vi "AcquireImages.vi"(8 "Error In":errorcluster, 9 "Acquisition Parameters":T5={"Acquisition Mode"=enum."Single Scan", "Trigger Mode"=enum."Internal", "Frame \nTransfer"=FALSE, "Exposure Time (s)"=0.0, "Accumulation Cycle Time (s)"=0.0, "# Accumulations"=1, "# Kinetics"=1, "Kinetic Cycle Time (s)"=0.0, "Horizontal Bin Size"=1, "Vertical Bin Size"=1} {"Vertical Bin Size" min=1; "Horizontal Bin Size" min=1; "Kinetic Cycle Time (s)" format="%.2f"; "# Kinetics" min=1; "# Accumulations" min=1; "Accumulation Cycle Time (s)" format="%.2f"; "Exposure Time (s)" format="%.2e"}, 10 "Camera Information 2":T1 {"VS Speed (us)" format="%.2f"}, 11 "Pre Initialized?":bool) -> (0 "error out":errorcluster, 1 "Intensity Graph":i32[][](graph))   [LabVIEW 2013]
uses:
  camera_controls.ctl
  <userlib>/atmcd32d.llb/AcquisitionMode_mode typedef.ctl
  <userlib>/atmcd32d.llb/TriggerMode_mode typedef.ctl
  acquisition_states.ctl
  CameraTest/System Files/user.lib/atmcd32d.llb/Error Code Enum typedef.ctl
panel:
  out "Total Number Pixels":dbl format="%#_6f"
  out "Img Y Size":dbl
  out "Img X Size":dbl
  out "size(s)":i32[](array[numeric])
  out "# Acq'd Images":u32
  out "1D Images":i32[](array[numeric])
  out "Acq. Error Codes":T2
  out "Calcualted Times":T3 {"Kinetic" format="%.2f"; "Accumulate" format="%.2f"; "Exposure" format="%.2f"}
  out "Andor Initialization Error Codes":T4
  out "Camera Information":T1 {"VS Speed (us)" format="%.2f"}
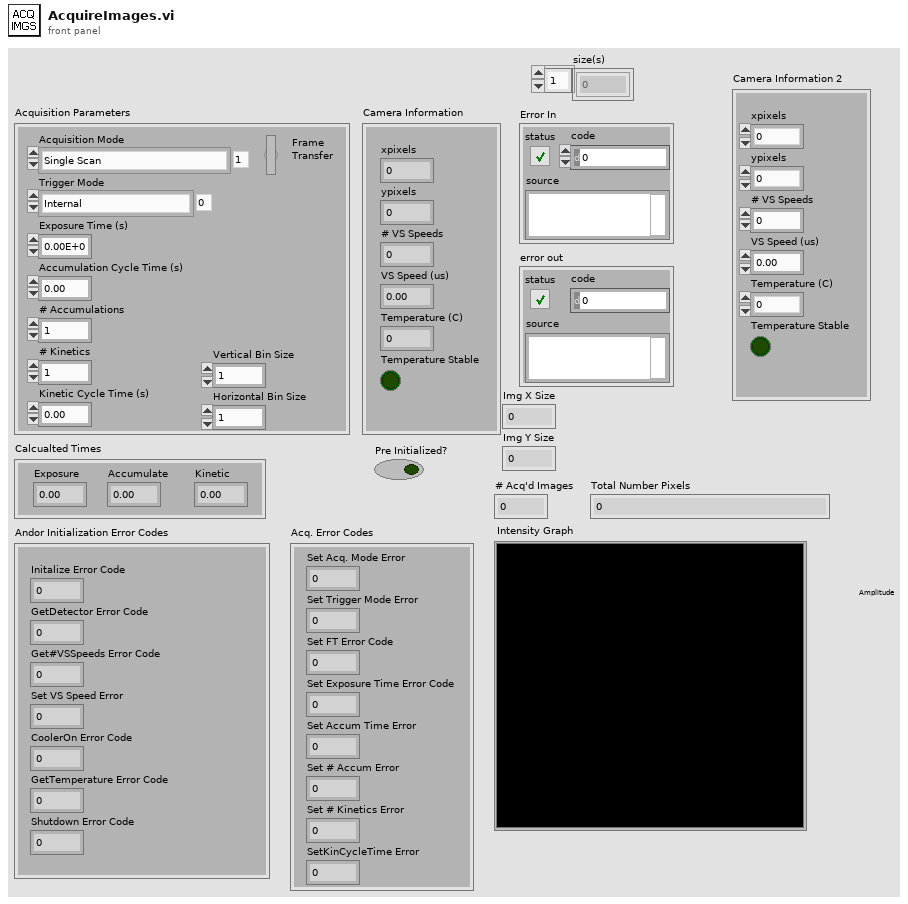
[diagram p1: front panel]
types:
  T1 = cluster{"xpixels":i32, "ypixels":i32, "# VS Speeds":i32, "VS Speed (us)":sgl, "Temperature Stable":bool, "Temperature (C)":i32}
  T2 = cluster{"Set Acq. Mode Error":u32, "Set Trigger Mode Error":u32, "Set FT Error Code":u32, "Set Exposure Time Error Code":u32, "Set Accum Time Error":u32, "Set # Accum Error":u32, "Set # Kinetics Error":u32, "SetKinCycleTime Error":u32}
  T3 = cluster{"Exposure":sgl, "Accumulate":sgl, "Kinetic":sgl}
  T4 = cluster{"Initalize Error Code":u32, "GetDetector Error Code":u32, "Get#VSSpeeds Error Code":u32, "Set VS Speed Error":u32, "CoolerOn Error Code":u32, "GetTemperature Error Code":u32, "Shutdown Error Code":u32}
  T5 = typedef "camera_controls.ctl" = cluster{"Acquisition Mode":T6, "Trigger Mode":T7, "Frame \nTransfer":bool, "Exposure Time (s)":sgl, "Accumulation Cycle Time (s)":sgl, "# Accumulations":i32, "# Kinetics":i32, "Kinetic Cycle Time (s)":sgl, "Horizontal Bin Size":i32, "Vertical Bin Size":i32}
  T6 = typedef "AcquisitionMode_mode typedef.ctl" = enum16{"Reserved (0)", "Single Scan", "Accumulate", "Kinetics", "Fast Kinetics", "Run Till Abort", "Reserved (6)", "Reserved (7)", "Reserved (8)", "Time Delayed Integration"}
  T7 = typedef "TriggerMode_mode typedef.ctl" = enum16{"Internal", "External", "N/A (2)", "N/A (3)", "N/A (4)", "N/A (5)", "External Start", "External Exposure (Bulb)", "N/A (8)", "External FVB EM", "Software", "N/A (11)", "External Charge Shifting"}
  T8 = typedef "acquisition_states.ctl" = enum16{"Initialize", "Set Params", "Begin Acquisition", "Retrive Data", "Display Data"}
  T9 = typedef "Error Code Enum typedef.ctl" = enum32{"N/A (0)", "DRV_ERROR_CODES", "DRV_SUCCESS", "DRV_VXDNOTINSTALLED", "DRV_ERROR_SCAN", "DRV_ERROR_CHECK_SUM", "DRV_ERROR_FILELOAD", "DRV_UNKNOWN_FUNC", "DRV_ERROR_VXD_INIT", "DRV_ERROR_ADDRESS", "DRV_ERROR_PAGELOCK", "DRV_ERROR_PAGEUNLOCK", "DRV_ERROR_BOARDTEST", "DRV_ERROR_ACK", "DRV_ERROR_UP_FIFO", "DRV_ERROR_PATTERN", "N/A (16)", "DRV_ACQUISITION_ERRORS", "DRV_ACQ_BUFFER", "DRV_ACQ_DOWNFIFO_FULL", "DRV_PROC_UNKONWN_INSTRUCTION", "DRV_ILLEGAL_OP_CODE", "DRV_KINETIC_TIME_NOT_MET", "DRV_ACCUM_TIME_NOT_MET", "DRV_NO_NEW_DATA", "N/A (25)", "DRV_SPOOLERROR", "N/A (27)", "N/A (28)", "N/A (29)", "N/A (30)", "N/A (31)", "N/A (32)", "DRV_TEMPERATURE_CODES", "DRV_TEMPERATURE_OFF", "DRV_TEMPERATURE_NOT_STABILIZED", "DRV_TEMPERATURE_STABILIZED", "DRV_TEMPERATURE_NOT_REACHED", "DRV_TEMPERATURE_OUT_RANGE", "DRV_TEMPERATURE_NOT_SUPPORTED", "DRV_TEMPERATURE_DRIFT", "N/A (41)", "N/A (42)", "N/A (43)", "N/A (44)", "N/A (45)", "N/A (46)", "N/A (47)", "N/A (48)", "DRV_GENERAL_ERRORS", "DRV_INVALID_AUX", "DRV_COF_NOTLOADED", "DRV_FPGAPROG", "DRV_FLEXERROR", "DRV_GPIBERROR", "N/A (55)", "N/A (56)", "N/A (57)", "N/A (58)", "N/A (59)", "N/A (60)", "N/A (61)", "N/A (62)", "N/A (63)", "DRV_DATATYPE", "DRV_DRIVER_ERRORS", "DRV_P1INVALID", "DRV_P2INVALID", "DRV_P3INVALID", "DRV_P4INVALID", "DRV_INIERROR", "DRV_COFERROR", "DRV_ACQUIRING", "DRV_IDLE", "DRV_TEMPCYCLE", "DRV_NOT_INITIALIZED", "DRV_P5INVALID", "DRV_P6INVALID", "DRV_INVALID_MODE", "DRV_INVALID_FILTER", "DRV_I2CERRORS", "DRV_I2CDEVNOTFOUND", "DRV_I2CTIMEOUT", "DRV_P7INVALID", "N/A (84)", "N/A (85)", "N/A (86)", "N/A (87)", "N/A (88)", "N/A (89)", "DRV_IOCERROR", "DRV_VRMVERSIONERROR"}
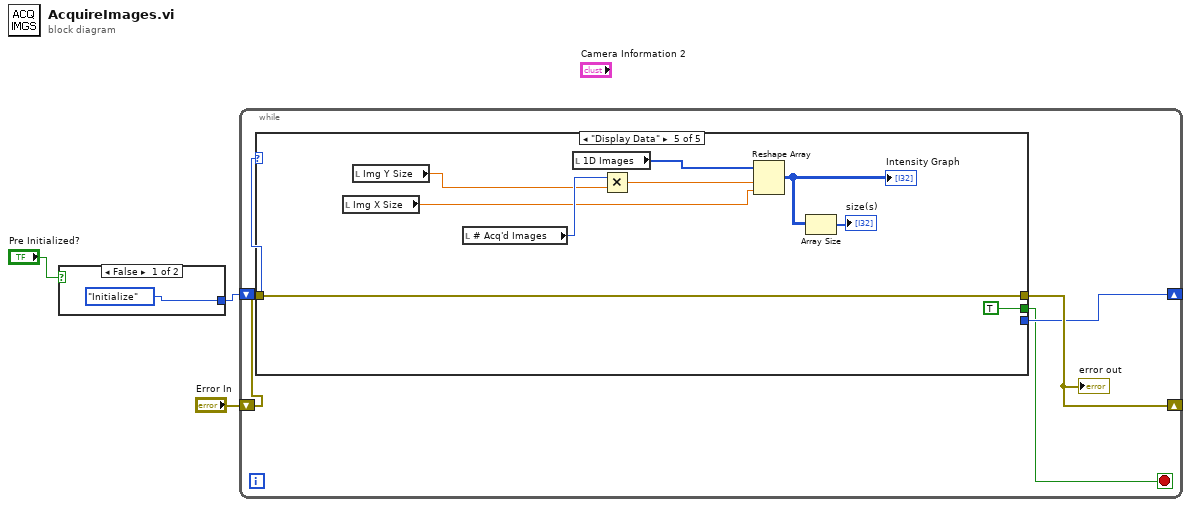
[diagram p0: block diagram]
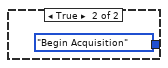
[diagram p2: hidden frame]
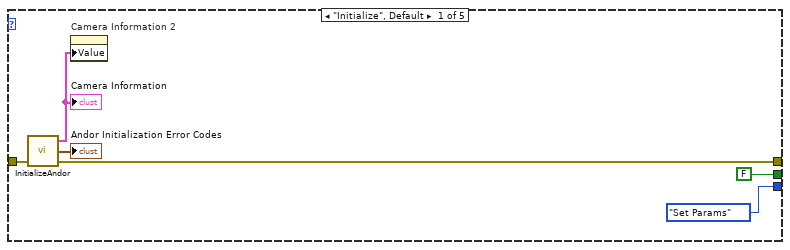
[diagram p3: hidden frame]
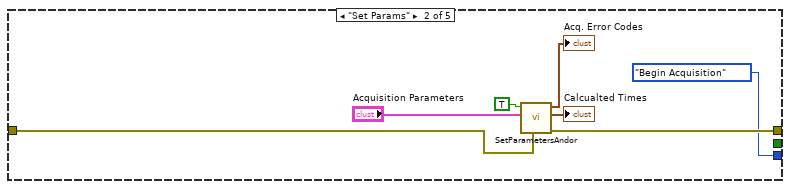
[diagram p4: hidden frame]
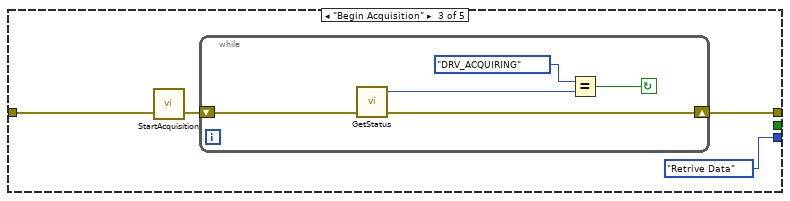
[diagram p5: hidden frame]
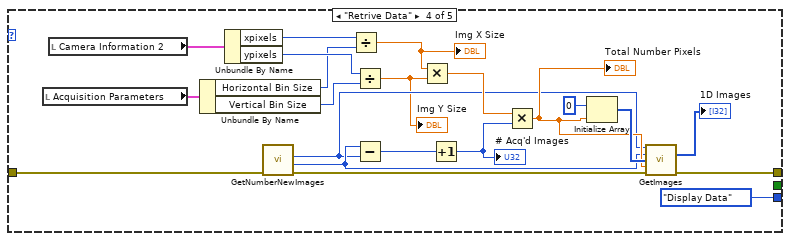
[diagram p6: hidden frame]
diagram:
  n1 = case shown="False" "Pre Initialized?" {
    tunnel: [acquisition_states."Initialize" acquisition_states."Begin Acquisition"] -> w3
    frame False {
    }
    frame True {
    }
  }
  n2 = while {
    shift-right: [w8] -> _
    shift-left: "Error In" -> [w9]
    shift-right: [w7] -> _
    shift-left: w3 -> [w10]
    stop <- w6 stop-if-true
    n3 = case shown="\"Display Data\"" w10 {
      tunnel: w9 -> [w16 w21 w27 w53 w60]
      tunnel: [w15 w20 w25 w47 w60] -> w8
      tunnel: [acquisition_states."Set Params" acquisition_states."Begin Acquisition" acquisition_states."Retrive Data" acquisition_states."Display Data" _] -> w7
      tunnel: [FALSE _ _ _ TRUE] -> w6
      frame "Initialize", Default {
        n4 = call "InitializeAndor.vi"("Error In"=w16) -> ("error out"=w15:errorcluster, "Andor Initialization Error Codes"=→"Andor Initialization Error Codes":T4, "Camera Information"=w11:T1)  [unwired: 2 in]
        "Camera Information" <- w11
        n5 = property on="Camera Information 2" class="Clust (strict)"("Value"=w11) -> ()  [unwired: 2 in, 2 out]
      }
      frame "Set Params" {
        n6 = call "SetParametersAndor.vi"("Error In"=w21, "Acquisition Parameters"="Acquisition Parameters", "Pre Initialized?"=TRUE) -> ("error out"=w20:errorcluster, "Calcualted Times"=→"Calcualted Times":T3, "Acq. Error Codes"=→"Acq. Error Codes":T2)  [unwired: 6 in]
      }
      frame "Begin Acquisition" {
        n7 = call <userlib>:"StartAcquisition.vi"("error in (no error)"=w27) -> ("error out"=w26:errorcluster)  [unwired: 1 in, 1 out]
        n8 = while {
          shift-right: [w28] -> w25
          shift-left: w26 -> [w32]
          stop <- w29 continue-if-true
          n9 = call <userlib>:"GetStatus.vi"("error in (no error)"=w32) -> ("error out"=w28:errorcluster, "status"=w31:T9)  [unwired: 2 in, 1 out]
          n10 = Equal?(x=Error_Code_Enum_typedef."DRV_ACQUIRING", y=w31) -> (x = y?=w29:bool)
        }
      }
      frame "Retrive Data" {
        n11 = local read "Acquisition Parameters"() -> (w39:T5)
        n12 = local read "Camera Information 2"() -> (w40:T1)
        n13 = Unbundle By Name(w39) -> ("Horizontal Bin Size"=w34:i32, "Vertical Bin Size"=w37:i32)
        n14 = Unbundle By Name(w40) -> ("xpixels"=w35:i32, "ypixels"=w38:i32)
        n15 = call <userlib>:"GetNumberNewImages.vi"("error in (no error)"=w53) -> ("error out"=w48:errorcluster, "last"=w42:i32, "first"=w41:u32)  [unwired: 3 in, 1 out]
        n16 = Divide(x=w35, y=w34) -> (x/y=w33:dbl)
        "Img X Size" <- w33
        n17 = Divide(x=w38, y=w37) -> (x/y=w36:dbl)
        "Img Y Size" <- w36
        n18 = Subtract(x=w42, y=w41) -> (x-y=w44:u32)
        n19 = Multiply(x=w33, y=w36) -> (x*y=w51:dbl)
        n20 = Increment(x=w44) -> (x+1=w43:u32)
        "# Acq'd Images" <- w43
        n21 = Multiply(x=w51, y=w43) -> (x*y=w49:dbl)
        "Total Number Pixels" <- w49
        n22 = Initialize Array(0, w49) -> (w50:i32[])
        n23 = call <userlib>:"GetImages.vi"("first"=w41, "last"=w42, "array"=w50, "size"=w49, "error in (no error)"=w48) -> ("array"=→"1D Images":i32[], "error out"=w47:errorcluster)  [unwired: 6 in, 3 out]
      }
      frame "Display Data" {
        n24 = local read "Img X Size"() -> (w56:dbl)
        n25 = local read "Img Y Size"() -> (w58:dbl)
        n26 = local read "# Acq'd Images"() -> (w62:u32)
        n27 = local read "1D Images"() -> (w54:i32[])
        n28 = Multiply(x=w62, y=w58) -> (x*y=w55:dbl)
        n29 = Reshape Array(w54, w55, w56) -> (w57:i32[][])
        "Intensity Graph" <- w57
        n30 = Array Size(array=w57) -> (size(s)=→"size(s)":i32[])
      }
    }
    "error out" <- w8
  }
